vi "Fetch DateTime data.vi"(4 "error in (no error)":errorcluster, 7 "Statement Refnum":T1) -> (0 "error out":errorcluster, 2 "Data":timestamp, 3 "Statement Refnum":T1)   [LabVIEW 2011]
doc: "Lit la donnée de type DateHeure (format string)"
uses:
  SQL Controls/Statement Refnum.ctl
  Odbc32.dll
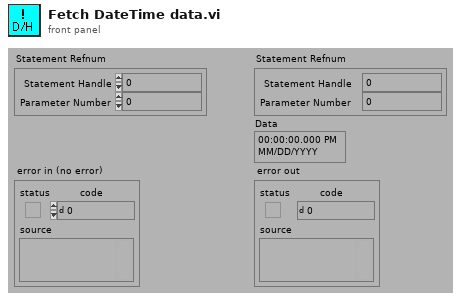
[diagram p1: front panel]
types:
  T1 = typedef "Statement Refnum.ctl" = cluster{"Statement Handle":i32, "Parameter Number":u16}
  T2 = enum16{"NOPE", "SQL_HANDLE_ENV", "SQL_HANDLE_DBC", "SQL_HANDLE_STMT", "SQL_HANDLE_DESC"}
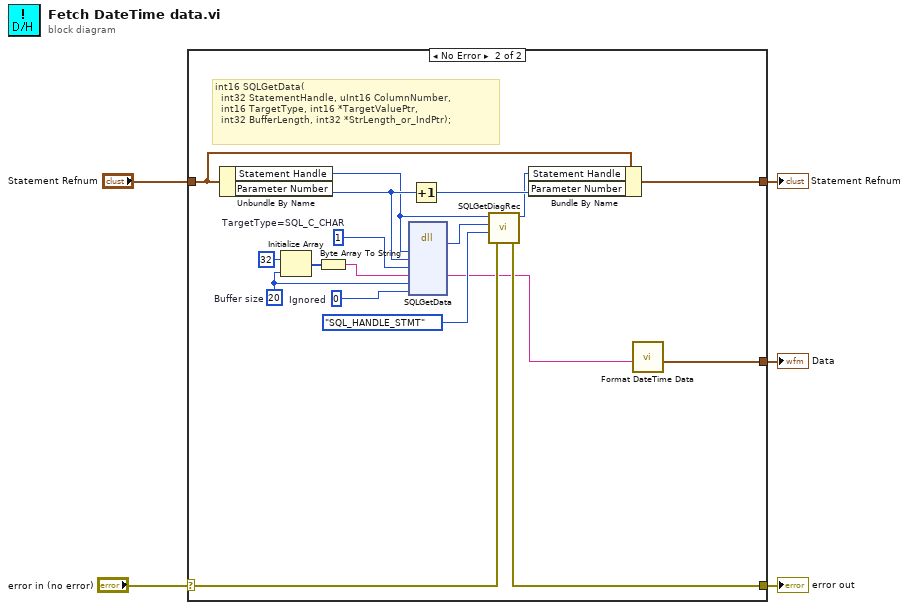
[diagram p0: block diagram]
diagram:
  n1 = case shown="No Error" "error in (no error)" {
    selector: "error in (no error)" -> [w6 w10]
    tunnel: "Statement Refnum" -> [w7 w19]
    tunnel: [w7 w18] -> w4
    tunnel: [w6 w12] -> w3
    tunnel: [_ w8] -> w2
    frame Error {
    }
    frame No Error {
      w24 = i16 1  # TargetType=SQL_C_CHAR
      w23 = 20  # Buffer size
      w25 = 0  # Ignored
      # "int16 SQLGetData(\n  int32 StatementHandle, uInt16 ColumnNumber, \n  int16 TargetType, int16 *TargetValuePtr,\n  int32 BufferLength, int32 *StrLength_or_IndPtr);"
      n2 = Unbundle By Name(w19) -> ("Statement Handle"=w15:i32, "Parameter Number"=w16:u16)
      n3 = Initialize Array(u8 32, w23) -> (w21:u8[])
      n4 = Byte Array To String(unsigned byte array=w21) -> (string=w20:string)
      n5 = dll-call lib="Odbc32.dll" fn="SQLGetData"("StatementHandle"=w15, "ColumnNumber"=w16, "TargetType"=w24, "TargetValuePtr"=w20, "BufferLength"=w23, "StrLength_or_IndPtr"=w25) -> (w14:i16, "TargetValuePtr"=w9:string)  [unwired: 7 in, 3 out]
      n6 = Increment(x=w16) -> (x+1=w17:u16)
      n7 = call "SQLGetDiagRec.vi"("error in (no error)"=w10, "HandleType"=T2."SQL_HANDLE_STMT", "Status (SQL_SUCCESS=0)"=w14, "Input Handle"=w15) -> ("error out"=w12:errorcluster, "Output Handle"=w11:i32)  [unwired: 2 out]
      n8 = Bundle By Name(cluster=w19, "Statement Handle"=w11, "Parameter Number"=w17) -> (w18:T1)
      n9 = call "Format DateTime Data.vi"("DB String in"=w9) -> ("Timestamp out"=w8:timestamp)  [unwired: 10 out]
    }
  }
  "error out" <- w3
  "Statement Refnum" <- w4
  "Data" <- w2
